vi "UPnPgetServerName.vi"() -> (3 "ServerName":string)   [LabVIEW 2010]
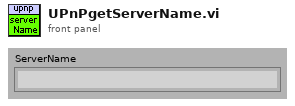
[diagram p1: front panel]
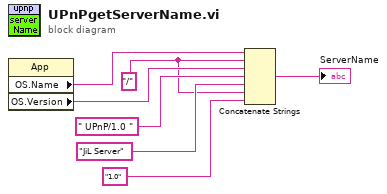
[diagram p0: block diagram]
diagram:
  w1 = "/" ("string")
  n1 = property class="App"() -> ("OS.Name"=w7:string, "OS.Version"=w5:string)  [unwired: 2 in, 2 out]
  n2 = Concatenate Strings(w7, w1, w5, " UPnP/1.0 " ("string"), "JiL Server" ("string"), w1, "1.0" ("string")) -> (→"ServerName":string)
